vi "OVA_SetWLCtrlLimits.vi"(5 "Wavelength Range (nm)":refnum<vi>, 6 "Center WL (nm)":refnum<vi>) -> ()   [LabVIEW 2024]
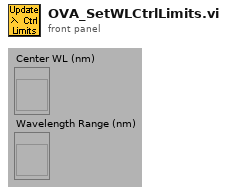
[diagram p1: front panel]
types:
  T1 = cluster{"calStartWL":dbl, "avgs":u32, "timeLength":dbl, "deciFactor":u32, "minStartWL":dbl, "rangeArray":dbl[], "minAvgs":u32, "maxAvgs":u32, "measType":u8, "timeStamp":string, "dutLength":dbl}
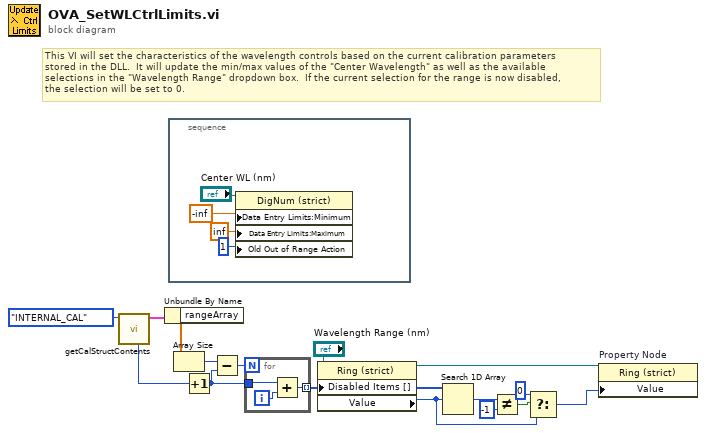
[diagram p0: block diagram]
diagram:
  # "This VI will set the characteristics of the wavelength controls based on the current calibration parameters\nstored in the DLL.  It will update the min/max values of the \"Center Wavelength\" as well as the available \nselections in the \"Wavelength Range\" dropdown box.  If the current selection for the range is now disabled,\nthe selection will be set to 0."
  n1 = call "getCalStructContents.vi"("calType"=enum16{"INTERNAL_CAL", "FULL_CAL"}."INTERNAL_CAL") -> ("Calibration Information"=w16:T1, "Range Selection"=w13:i32)  [unwired: 7 in, 2 out]
  n2 = Unbundle By Name(w16) -> ("rangeArray"=w15:dbl[])
  n3 = stacked-sequence {
    frame #0 {
      n4 = property class="DigNum (strict)"(reference="Center WL (nm)", "Data Entry Limits:Minimum"=-inf ("Data Range:Minimum"), "Data Entry Limits:Maximum"=inf ("Data Range:Maximum"), "Old Out of Range Action"=u8 1 ("Out of Range Action")) -> ()  [unwired: 1 in, 2 out]
    }
  }
  n5 = Array Size(array=w15) -> (size(s)=w14:i32)
  n6 = Increment(x=w13) -> (x+1=w12:i32)
  n7 = Subtract(x=w14, y=w12) -> (x-y=w11:i32)
  n8 = for {
    N: w11 -> [_]
    tunnel: w12 -> [w22]
    tunnel: [w21] -> w10 mode=indexing
    i -> [w23]
    n9 = Add(x=w22, y=w23) -> (x+y=w21:i32)
  }
  n10 = property class="Ring (strict)"(reference="Wavelength Range (nm)", "Disabled Items []"=w10) -> (reference out=w8:refnum<vi>, "Value"=w4:u16)  [unwired: 1 in, 1 out]
  n11 = Search 1D Array(1D array=w10, element=w4) -> (index of element=w7:i32)  [unwired: 1 in]
  n12 = Not Equal?(x=w7, y=-1) -> (x != y?=w5:bool)
  n13 = Select(t=0, s=w5, f=w4) -> (s? t:f=w2:i32)
  n14 = property on="Property Node" class="Ring (strict)"(reference=w8, "Value"=w2) -> ()  [unwired: 1 in, 2 out]
